vi "Test Energy and Pulse Calculation.vi"(3 "Capacitor Size (f)":dbl=6.23e-06, 4 "Max Test Voltage (V)":dbl format="%#_3p", 5 "Stick Energy (J)":dbl format="%#_3p") -> (0 "Actual Test Voltage (V)":dbl format="%#_4p", 1 "Actual No. of Pulses":i32, 2 "Actual Pulse Energy (J)":dbl format="%#_4p")   [LabVIEW 2015]
panel:
  out "Total Actual Energy (J)":dbl format="%#_3p"
  out "Requested No. of Pulses":dbl format="%#_4p"
  out "Max Pulse Energy (J)":dbl format="%#_3p"
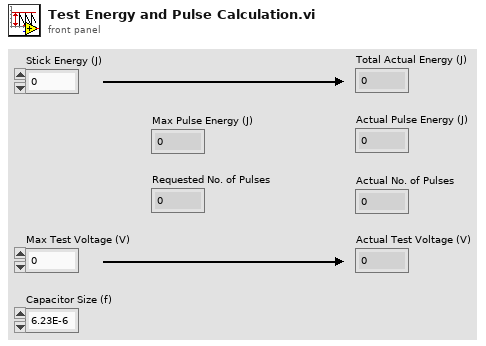
[diagram p1: front panel]
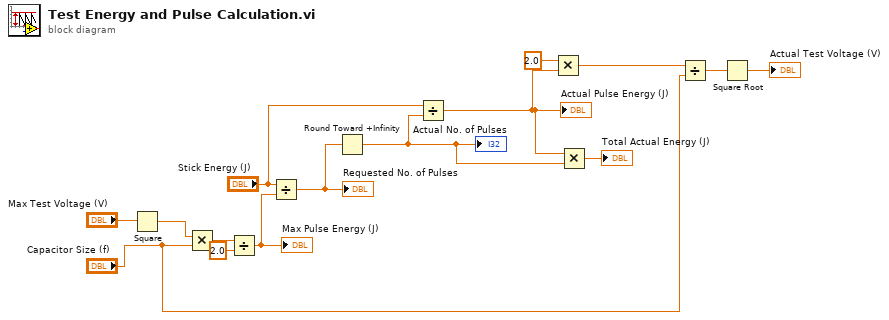
[diagram p0: block diagram]
diagram:
  n1 = Square(x="Max Test Voltage (V)") -> (x^2=w14:dbl)
  n2 = Multiply(x=w14, y="Capacitor Size (f)") -> (x*y=w13:dbl)
  n3 = Divide(x=w13, y=2.0) -> (x/y=w11:dbl)
  "Max Pulse Energy (J)" <- w11
  n4 = Divide(x="Stick Energy (J)", y=w11) -> (x/y=w10:dbl)
  "Requested No. of Pulses" <- w10
  n5 = Round Toward +Infinity(x=w10) -> (ceil(x): smallest int >= x=w2:dbl)
  "Actual No. of Pulses" <- w2
  n6 = Divide(x="Stick Energy (J)", y=w2) -> (x/y=w3:dbl)
  "Actual Pulse Energy (J)" <- w3
  n7 = Multiply(x=2.0, y=w3) -> (x*y=w7:dbl)
  n8 = Multiply(x=w3, y=w2) -> (x*y=→"Total Actual Energy (J)":dbl)
  n9 = Divide(x=w7, y="Capacitor Size (f)") -> (x/y=w5:dbl)
  n10 = Square Root(x=w5) -> (sqrt(x)=→"Actual Test Voltage (V)":dbl)
